vi "Create File Response.vi"   [LabVIEW 2020]
uses:
  lv-http-util/HTTP Utils/File Response/File Response.lvclass
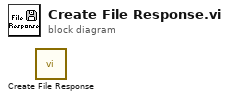
[diagram p0: block diagram]
diagram:
  n1 = call "Create File Response.vi"() -> ()  [unwired: 10 in, 2 out]
